vi "IMU_Viewer.vi"() -> ()   [LabVIEW 2011]
uses:
  <vilib>/Instr/_visa.llb/VISA Flush IO Buffer Mask.ctl
  <vilib>/Instr/_visa.llb/VISA Configure Serial Port (Instr).vi
  <vilib>/express/express arith-compare/Formula/XNode/ExpressFormulaBlockNode.xnode
  <vilib>/picture/3D Picture Control/NI_3D Picture Control.lvlib
panel:
  out "Kompass":dbl(knob) caption="Gauge 2" scale=0.0..360.0
  out "Magnetometer RAW":cluster{"Mx":sgl, "My":sgl, "Mz":sgl}(graph)
  out "Gyroscope RAW":cluster{"Gx":sgl, "Gy":sgl, "Gz":sgl}(graph)
  out "Lesepuffer":string
  in  "GetData":bool
  out "Acceleration RAW":cluster{"Ax":sgl, "Ay":sgl, "Az":sgl}(graph)
  out "Cluster":T1
  out "Rotation":refnum<vi>(3d-picture)
  in  "VISA resource name":refnum<visa-resource-name> caption="VISA-Ressourcenname"
  out "Vergangene Zeit":timestamp
  in  "Stopp":bool
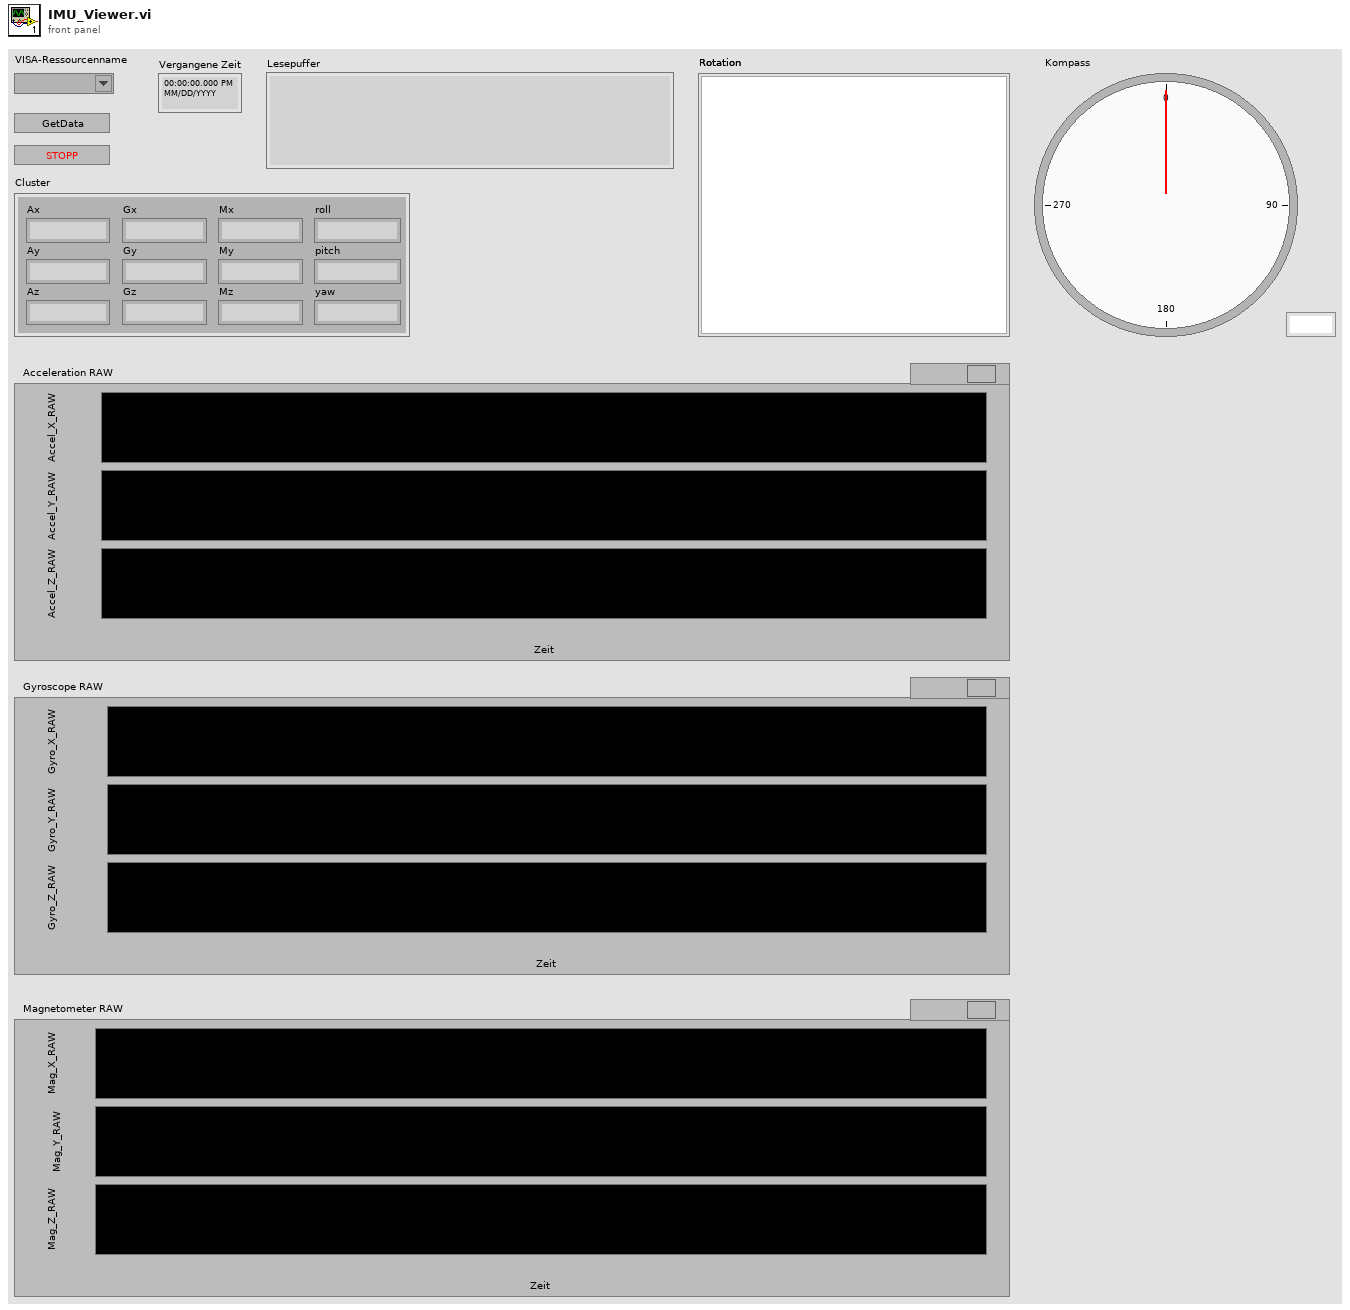
[diagram p1: front panel]
types:
  T1 = cluster{"Ax":sgl, "Ay":sgl, "Az":sgl, "Gx":sgl, "Gy":sgl, "Gz":sgl, "Mx":sgl, "My":sgl, "Mz":sgl, "roll":sgl, "pitch":sgl, "yaw":sgl}
  T2 = typedef "VISA Flush IO Buffer Mask.ctl" = u16
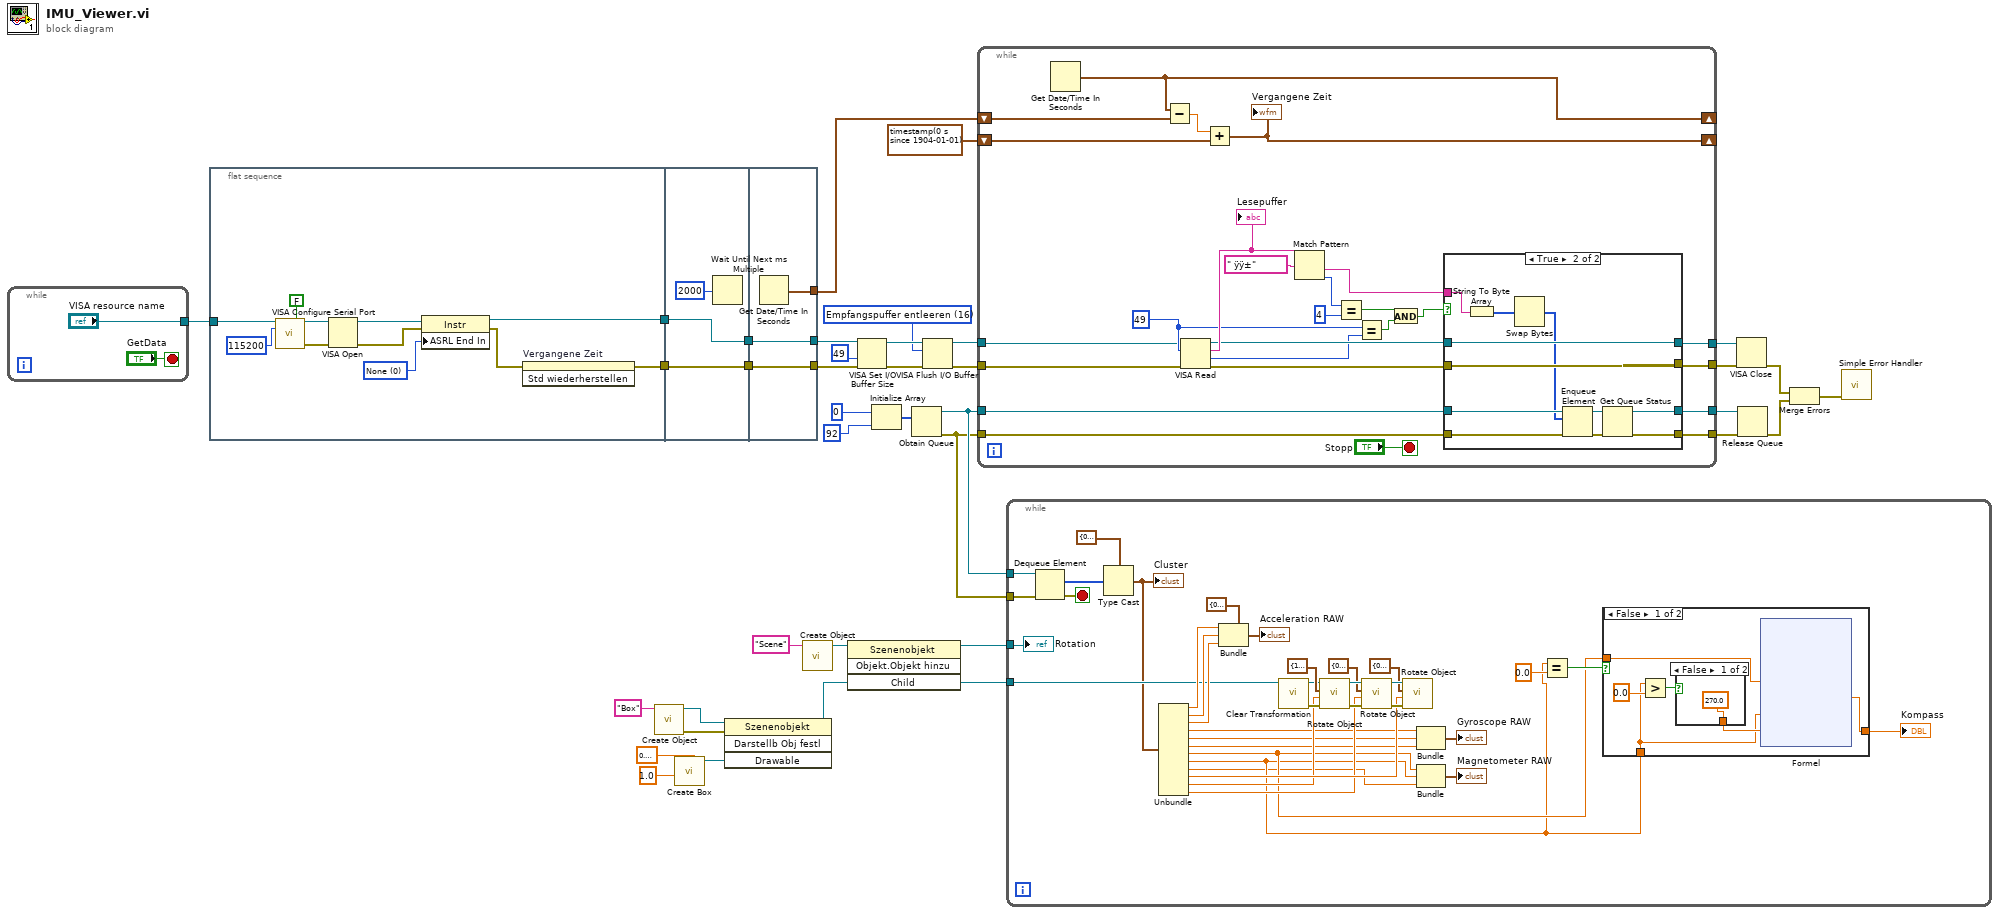
[diagram p0: block diagram]
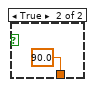
[diagram p2: hidden frame]
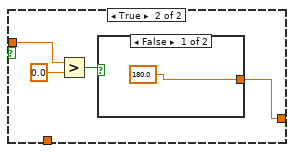
[diagram p3: hidden frame]
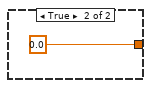
[diagram p4: hidden frame]
diagram:
  w5 = T2 16 items=["Empfangspuffer entleeren"=16, "Übertragungspuffer in Gerät schreiben"=32, "Empfangspuffer entleeren (keine I/O)"=64, "Übertragungspuffer entleeren"=128] ("Mask")
  w13 = sgl 1.0 ("Length Y")
  n1 = while {
    tunnel: ["VISA resource name"] -> w10
    stop <- "GetData" stop-if-true
  }
  n2 = flat-sequence {
    tunnel: [w42] -> w12
    tunnel: [w43] -> w11
    tunnel: w10 -> [w41]
    tunnel: [w52] -> w29
    tunnel: [w53] -> w28
    tunnel: w12 -> [w53]
    tunnel: w11 -> [w52]
    tunnel: [w57] -> w38
    tunnel: [w56] -> w16
    tunnel: w29 -> [w56]
    tunnel: [w55] -> w15
    tunnel: w28 -> [w55]
    frame #0 {
      w45 = u16 0 items=["None", "Last Bit", "TermChar"] ("Serial Settings:End Mode for Reads")
      n3 = call-poly "VISA Configure Serial Port"("VISA resource name"=w41, "Enable Termination\nChar (T)"=FALSE ("Enable Termination\nChar (T)"), "baud rate (9600)"=u32 115200) -> ("VISA resource name out"=w50:refnum<visa-resource-name>, "error out"=w51:errorcluster)  [unwired: 11 in]
      n4 = VISA Open(error in (no error)=w51, VISA resource name=w50) -> (VISA resource name=w49:refnum<visa-resource-name>, error out=w48:errorcluster)  [unwired: 3 in]
      n5 = property class="Instr"(reference=w49, error in=w48, "ASRL End In"=w45) -> (reference out=w43:refnum<visa-resource-name>, error out=w46:errorcluster)
      n6 = invoke on="Vergangene Zeit" class="AbsZeit (strikt)" method="Std wiederherstellen"(error in=w46) -> (error out=w42:errorcluster)  [unwired: 2 in, 2 out]
    }
    frame #1 {
      n7 = Wait Until Next ms Multiple(millisecond multiple=u32 2000 ("Vielfache von ms")) -> ()  [unwired: 1 out]
    }
    frame #2 {
      n8 = Get Date/Time In Seconds() -> (seconds since 1Jan1904=w57:timestamp)
    }
  }
  n9 = call <vilib>:"Create Object.vi"("Name"="Box") -> ("error out"=w22:errorcluster, "Scene:New Object"=w27:refnum<vi>)  [unwired: 9 in]
  n10 = call <vilib>:"Create Box.vi"("Length Z"=w13, "Length Y"=sgl 0.2 ("Length X"), "Length X"=w13) -> ("New Box Refnum"=w4:refnum<vi>)  [unwired: 7 in, 1 out]
  n11 = invoke class="Szenenobjekt" method="Darstellb Obj festl"(reference=w27, error in=w22, "Drawable"=w4) -> (reference out=w1:refnum<vi>)  [unwired: 1 in, 3 out]
  n12 = call <vilib>:"Create Object.vi"("Name"="Scene") -> ("Scene:New Object"=w2:refnum<vi>)  [unwired: 9 in, 1 out]
  n13 = invoke class="Szenenobjekt" method="Objekt.Objekt hinzu"(reference=w2, "Child"=w1) -> (reference out=w23:refnum<vi>, "Child"=w24:refnum<vi>)  [unwired: 2 in, 2 out]
  n14 = VISA Set I/O Buffer Size(VISA resource name=w16, size (4096)=u32 49 ("Größe (4096)"), error in (no error)=w15) -> (VISA resource name out=w6:refnum<visa-resource-name>, error out=w7:errorcluster)  [unwired: 1 in]
  n15 = Initialize Array(u8 0 ("Element"), 92 ("Dimension")) -> (w18:u8[])
  n16 = Obtain Queue(element data type=w18) -> (queue out=w26:refnum<queue>, error out=w25:errorcluster)  [unwired: 4 in, 1 out]
  n17 = VISA Flush I/O Buffer(VISA resource name=w6, mask (16)=w5, error in (no error)=w7) -> (VISA resource name out=w9:refnum<visa-resource-name>, error out=w8:errorcluster)
  n18 = while {
    shift-right: [w81] -> _
    shift-left: w38 -> [w82]
    shift-right: [w80] -> _
    shift-left: timestamp(0 s since 1904-01-01) ("seconds since 1Jan1904") -> [w66]
    tunnel: [w70] -> w36
    tunnel: [w68] -> w35
    tunnel: [w79] -> w34
    tunnel: [w78] -> w30
    tunnel: w26 -> [w76]
    tunnel: w25 -> [w77]
    tunnel: w8 -> [w59]
    tunnel: w9 -> [w60]
    stop <- "Stopp" stop-if-true
    w62 = u32 49 ("Byte-Anzahl")
    n19 = Get Date/Time In Seconds() -> (seconds since 1Jan1904=w81:timestamp)
    n20 = Subtract(x=w81, y=w82) -> (x-y=w67:dbl)
    n21 = VISA Read(VISA resource name=w60, byte count=w62, error in (no error)=w59) -> (VISA resource name out=w71:refnum<visa-resource-name>, read buffer=w74:string, return count=w61:u32, error out=w69:errorcluster)
    "Lesepuffer" <- w74
    n22 = Add(x=w67, y=w66) -> (x+y=w80:timestamp)
    "Vergangene Zeit" <- w80
    n23 = Match Pattern(string=w74, regular expression=" ÿÿ±" ("Regulärer Ausdruck")) -> (after substring=w58:string, offset past match=w73:i32)  [unwired: 1 in, 2 out]
    n24 = Equal?(x=w73, y=4) -> (x = y?=w65:bool)
    n25 = Equal?(x=w62, y=w61) -> (x = y?=w63:bool)
    n26 = And(x=w65, y=w63) -> (x .and. y?=w64:bool)
    n27 = case shown="True" w64 {
      tunnel: [w85 w92] -> w79
      tunnel: [w84 w93] -> w78
      tunnel: w77 -> [w84 w98]
      tunnel: w76 -> [w85 w97]
      tunnel: w71 -> [w87 w96]
      tunnel: [w87 w96] -> w70
      tunnel: w69 -> [w86 w95]
      tunnel: [w86 w95] -> w68
      tunnel: w58 -> [_ w90]
      frame False {
      }
      frame True {
        n28 = String To Byte Array(string=w90) -> (unsigned byte array=w89:u8[])
        n29 = Swap Bytes(anything=w89) -> (byte swapped=w88:u8[])
        n30 = Enqueue Element(queue=w97, element=w88, error in (no error)=w98) -> (queue out=w91:refnum<queue>, error out=w94:errorcluster)  [unwired: 1 in, 1 out]
        n31 = Get Queue Status(queue=w91, error in (no error)=w94) -> (queue out=w92:refnum<queue>, error out=w93:errorcluster)  [unwired: 1 in, 6 out]
      }
    }
  }
  n32 = while {
    tunnel: w25 -> [w134]
    tunnel: w26 -> [w133]
    tunnel: w24 -> [w114]
    tunnel: w23 -> [w131]
    stop <- w132 stop-if-true
    n33 = Dequeue Element(queue=w133, error in (no error)=w134) -> (element=w121:u8[], error out=w132:errorcluster)  [unwired: 1 in, 2 out]
    n34 = Type Cast(type=T1 {"Ax"=0.0, "Ay"=0.0, "Az"=0.0, "Gx"=0.0, "Gy"=0.0, "Gz"=0.0, "Mx"=0.0, "My"=0.0, "Mz"=0.0, "roll"=0.0, "pitch"=0.0, "yaw"=0.0} ("Cluster"), x=w121) -> (*(type *) &x=w109:T1)
    "Cluster" <- w109
    n35 = Unbundle(w109) -> ("Ax"=w117:sgl, "Ay"=w119:sgl, "Az"=w120:sgl, "Gx"=w104:sgl, "Gy"=w103:sgl, "Gz"=w102:sgl, "Mx"=w101:sgl, "My"=w100:sgl, "Mz"=w99:sgl, "roll"=w107:sgl, "pitch"=w106:sgl, "yaw"=w105:sgl)
    n36 = Bundle(cluster=cluster{"Ax":sgl, "Ay":sgl, "Az":sgl} {"Ax"=0.0, "Ay"=0.0, "Az"=0.0} ("Cluster"), "Ax"=w117, "Ay"=w119, "Az"=w120) -> (→"Acceleration RAW":cluster{"Ax":sgl, "Ay":sgl, "Az":sgl})
    n37 = call <vilib>:"Clear Transformation.vi"("Object Refnum In"=w114) -> ("error out"=w122:errorcluster, "Object Refnum Out"=w123:refnum<vi>)  [unwired: 9 in]
    n38 = call <vilib>:"Rotate Object.vi"("error in (no error)"=w122, "Angle"=w106, "Axis"=cluster{"X":sgl, "Y":sgl, "Z":sgl} {"X"=1.0, "Y"=0.0, "Z"=0.0}, "Scene.Object In"=w123) -> ("error out"=w125:errorcluster, "Scene.Object Out"=w130:refnum<vi>)  [unwired: 6 in]
    n39 = call <vilib>:"Rotate Object.vi"("error in (no error)"=w125, "Angle"=w105, "Axis"=cluster{"X":sgl, "Y":sgl, "Z":sgl} {"X"=0.0, "Y"=1.0, "Z"=0.0}, "Scene.Object In"=w130) -> ("error out"=w124:errorcluster, "Scene.Object Out"=w129:refnum<vi>)  [unwired: 6 in]
    n40 = call <vilib>:"Rotate Object.vi"("error in (no error)"=w124, "Angle"=w107, "Axis"=cluster{"X":sgl, "Y":sgl, "Z":sgl} {"X"=0.0, "Y"=0.0, "Z"=1.0}, "Scene.Object In"=w129) -> ()  [unwired: 6 in, 2 out]
    n41 = Bundle("Gx"=w104, "Gy"=w103, "Gz"=w102) -> (→"Gyroscope RAW":cluster{"Gx":sgl, "Gy":sgl, "Gz":sgl})  [unwired: 1 in]
    n42 = Bundle("Mx"=w101, "My"=w100, "Mz"=w99) -> (→"Magnetometer RAW":cluster{"Mx":sgl, "My":sgl, "Mz":sgl})  [unwired: 1 in]
    n43 = Equal?(x=w100, y=0.0) -> (x = y?=w113:bool)
    n44 = case shown="False" w113 {
      tunnel: w100 -> [w137 _]
      tunnel: w101 -> [w136 w156]
      tunnel: [w135 w155] -> w111
      frame False {
        n45 = Greater?(x=w137, y=0.0) -> (0:w140:bool)
        n46 = case shown="False" w140 {
          tunnel: [270.0 ("y") 90.0 ("y")] -> w138
          frame False {
          }
          frame True {
          }
        }
        n47 = xnode "Formel"("Mx"=w136, "My"=w137, "Base"=w138) -> ("Ergebnis"=w135:dbl)  [unwired: 1 in, 1 out]
      }
      frame True {
        n48 = Greater?(x=w156, y=0.0) -> (0:w158:bool)
        n49 = case shown="False" w158 {
          tunnel: [180.0 ("y") 0.0 ("y")] -> w155
          frame False {
          }
          frame True {
          }
        }
      }
    }
    "Kompass" <- w111
    "Rotation" <- w131
  }
  n50 = VISA Close(VISA resource name=w36, error in (no error)=w35) -> (error out=w33:errorcluster)
  n51 = Release Queue(queue=w34, error in (no error)=w30) -> (error out=w32:errorcluster)  [unwired: 1 in, 2 out]
  n52 = Merge Errors(w33, w32) -> (w31:errorcluster)
  n53 = call <vilib>:"Simple Error Handler.vi"("error in (no error)"=w31) -> ()  [unwired: 4 in, 5 out]
